vi "LD2018_ブロック崩し_BALL移動座標.vi"(9 "方向":i32, 10 "移動速度":dbl, 11 "角度":dbl) -> (3 "座標":cluster{dbl, dbl, dbl, dbl})   [LabVIEW 2017]
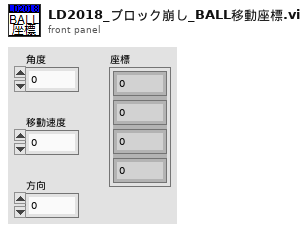
[diagram p1: front panel]
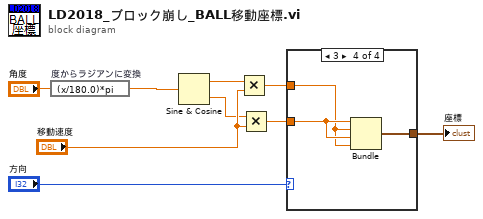
[diagram p0: block diagram]
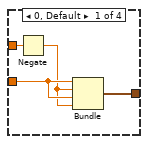
[diagram p2: hidden frame]
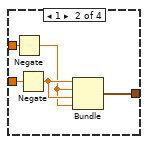
[diagram p3: hidden frame]
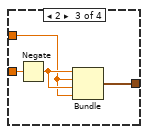
[diagram p4: hidden frame]
diagram:
  n1 = expression code="(x/180.0)*pi" "度からラジアンに変換"("角度") -> (w1:dbl)
  n2 = Sine & Cosine(0:w1) -> (1:w2:dbl, 2:w3:dbl)
  n3 = Multiply(x=w2, y="移動速度") -> (x*y=w5:dbl)
  n4 = Multiply(x=w3, y="移動速度") -> (x*y=w6:dbl)
  n5 = case shown="3" "方向" {
    tunnel: w5 -> [w13 w18 w19 w23]
    tunnel: w6 -> [w12 w17 w22 w24]
    tunnel: [w11 w15 w20 w25] -> w7
    frame 0, Default {
      n6 = Negate(x=w13) -> (-x=w10:dbl)
      n7 = Bundle(w12, w10, w12, w10) -> (w11:cluster{dbl, dbl, dbl, dbl})  [unwired: 1 in]
    }
    frame 1 {
      n8 = Negate(x=w18) -> (-x=w14:dbl)
      n9 = Negate(x=w17) -> (-x=w16:dbl)
      n10 = Bundle(w16, w14, w16, w14) -> (w15:cluster{dbl, dbl, dbl, dbl})  [unwired: 1 in]
    }
    frame 2 {
      n11 = Negate(x=w22) -> (-x=w21:dbl)
      n12 = Bundle(w21, w19, w21, w19) -> (w20:cluster{dbl, dbl, dbl, dbl})  [unwired: 1 in]
    }
    frame 3 {
      n13 = Bundle(w24, w23, w24, w23) -> (w25:cluster{dbl, dbl, dbl, dbl})  [unwired: 1 in]
    }
  }
  "座標" <- w7
